vi "DR200_control_B.vi"(7 "wait for  B?":bool, 8 "index":i32, 9 "set B (T)":dbl, 10 "sweep rate (T/min)":dbl, 11 "VISA resource name":refnum<visa-resource-name>="GPIB1::25::INSTR") -> (0 "Field (T)":dbl, 3 "VISA resource name":refnum<visa-resource-name>="GPIB1::25::INSTR")   [LabVIEW 2013]
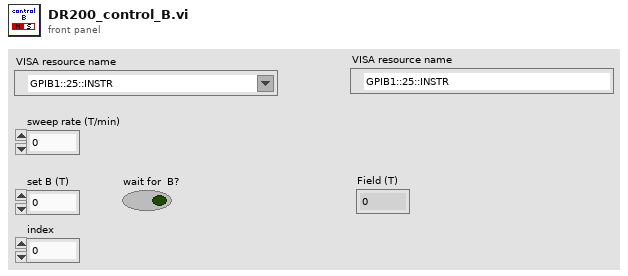
[diagram p1: front panel]
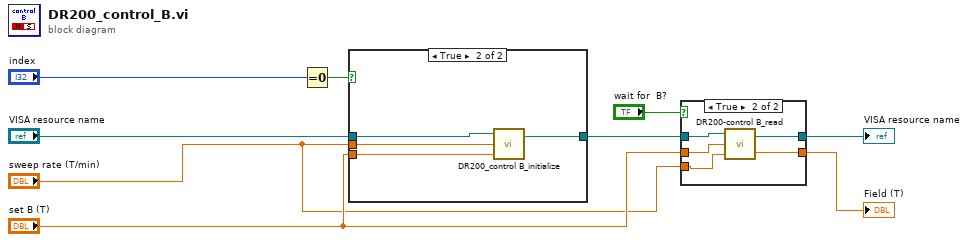
[diagram p0: block diagram]
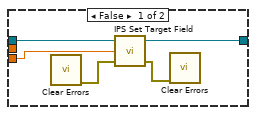
[diagram p3: hidden frame]
diagram:
  n1 = Equal To 0?(x="index") -> (x = 0?=w7:bool)
  n2 = case shown="True" w7 {
    tunnel: "VISA resource name" -> [w14 w18]
    tunnel: "set B (T)" -> [w13 w16]
    tunnel: [w12 w17] -> w5
    tunnel: "sweep rate (T/min)" -> [_ w15]
    frame False {
      n3 = call <vilib>:"Clear Errors.vi"() -> ("error out"=w11:errorcluster)  [unwired: 7 in]
      n4 = call "IPS Set Target Field.vi"("Error In"=w11, "Target Field (T)"=w13, "VISA resource name"=w14) -> ("Error Out"=w10:errorcluster, "VISA resource name"=w12:refnum<visa-resource-name>)  [unwired: 1 out]
      n5 = call <vilib>:"Clear Errors.vi"("error in (no error)"=w10) -> ()  [unwired: 6 in, 1 out]
    }
    frame True {
      n6 = call "DR200_control B_initialize.vi"("B set (T)"=w16, "Field Sweep Rate (T/min)"=w15, "VISA Refnum in"=w18) -> ("VISA Refnum out"=w17:refnum<visa-resource-name>)  [unwired: 1 in]
    }
  }
  n7 = case shown="True" "wait for  B?" {
    tunnel: w5 -> [w20 w25]
    tunnel: "set B (T)" -> [w19 w24]
    tunnel: [w20 w23] -> w3
    tunnel: [w19 w22] -> w2
    tunnel: "sweep rate (T/min)" -> [_ w21]
    frame False {
    }
    frame True {
      n8 = call "DR200-control B_read.vi"("sweep rate (T/min)"=w21, "set field (T)"=w24, "VISA Refnum in"=w25) -> ("Field (T)"=w22:dbl, "VISA resource name"=w23:refnum<visa-resource-name>)
    }
  }
  "VISA resource name" <- w3
  "Field (T)" <- w2
